vi "CTRE_CANifier_SetDeviceReference.vi"(8 "error in (no error)":errorcluster, 10 "refnum name":string="My CANifier RefNum", 11 "CANifierDevRef":T1) -> (0 "error out":errorcluster, 3 "CANifierDevRef":T1)   [LabVIEW 2017]
uses:
  CTRE_CANifier_DeviceRef.ctl
  <vilib>/Rock Robotics/WPI/Utilities/Refnum Registry Operation.ctl
panel:
  in  "Test Mode Only":bool
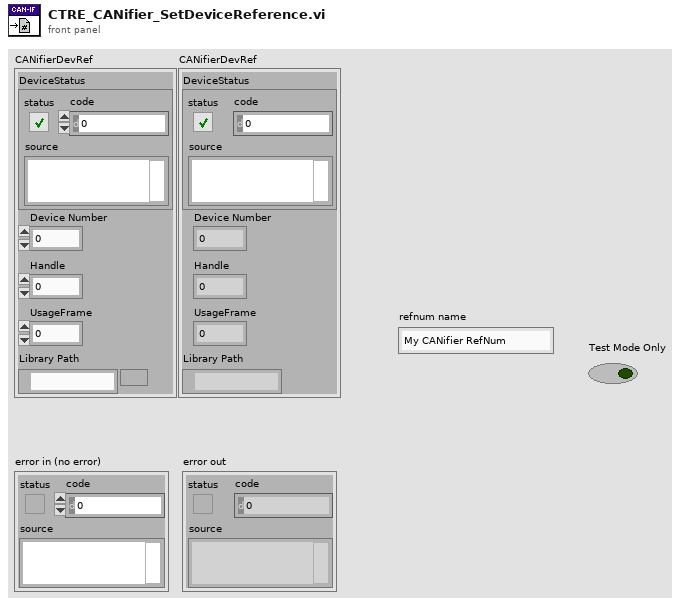
[diagram p1: front panel]
types:
  T1 = typedef "CTRE_CANifier_DeviceRef.ctl" = cluster{"DeviceStatus":errorcluster, "Device Number":u8, "Handle":u64, "UsageFrame":u32, "Library Path":path}
  T2 = typedef "Refnum Registry Operation.ctl" = enum16{"set", "get", "delete", "get all names", "read name"}
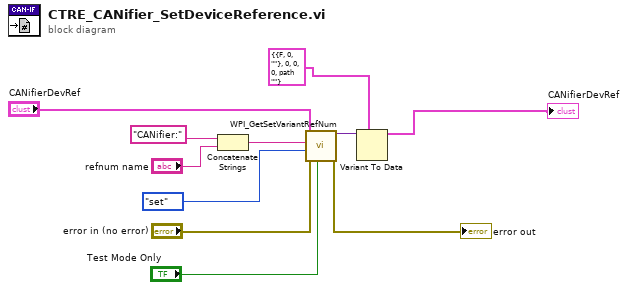
[diagram p0: block diagram]
diagram:
  n1 = Concatenate Strings("CANifier:", "refnum name") -> (w11:string)
  n2 = call <vilib>:"WPI_GetSetVariantRefNum.vi"("Test Mode Only"="Test Mode Only", "error in (no error)"="error in (no error)", "Operation"=Refnum_Registry_Operation."set" ("menu"), "refnum name"=w11, "DevRef"="CANifierDevRef") -> ("error out"=→"error out":errorcluster, "DevRef"=w9:variant)  [unwired: 4 in, 1 out]
  n3 = Variant To Data(type=T1 {"DeviceStatus"={"status"=FALSE, "code"=0, "source"=""}, "Device Number"=0, "Handle"=0, "UsageFrame"=0, "Library Path"=path ""} ("CANifierDevRef 3"), Variant=w9) -> (data=→"CANifierDevRef":T1)  [unwired: 1 in, 1 out]
